vi "Get Angle.vi"(8 "error in (no error)":errorcluster, 11 "Instrument.Oxford1820 in":refnum<class "Instrument.Oxford1820.lvclass">) -> (0 "error out":errorcluster, 1 "Status":variant, 2 "Angle (°)":dbl, 3 "Instrument.Oxford1820 out":refnum<class "Instrument.Oxford1820.lvclass">, 4 "Axis":T1)   [LabVIEW 2016, in "Instrument.Oxford1820.lvclass"]
uses:
  Instrument.Oxford1820.lvclass
  <userlib>/LevyLab/Levylab Instruments/Instrument Types/Cryostat/Typedefs/Rotator Axis--Enum.ctl
  <userlib>/LevyLab/Levylab Instruments/Instrument Types/Cryostat/Instrument.Cryostat.lvclass
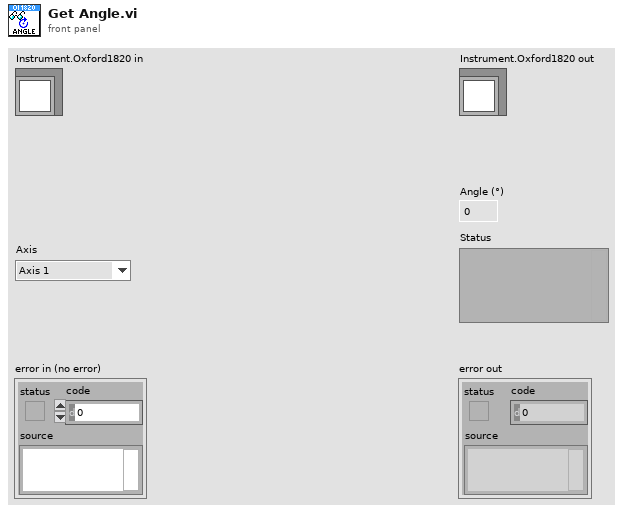
[diagram p1: front panel]
types:
  T1 = typedef "Instrument.Cryostat.lvclass/Rotator Axis--Enum.ctl" = enum16{"Axis 1", "Axis 2"}
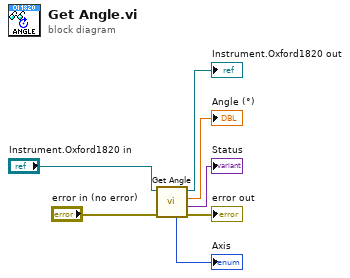
[diagram p0: block diagram]
diagram:
  n1 = call-parent "Get Angle.vi"("error in (no error)"="error in (no error)", "Instrument.Cryostat in"="Instrument.Oxford1820 in") -> ("error out"=→"error out":errorcluster, "Status"=→"Status":variant, "Angle (°)"=→"Angle (°)":dbl, "Instrument.Cryostat out"=→"Instrument.Oxford1820 out":refnum<class "Instrument.Oxford1820.lvclass">, "Axis"=→"Axis":T1)  [unwired: 5 in]
